vi "TimeLmtDialog.vi"(9 "time(s)":i32=5, 10 "Infoin":string="在这里填写显示的信息内容", 11 "title":string="提示信息") -> ()   [LabVIEW 2011]
panel:
  in  "ok":bool
  out "info":string
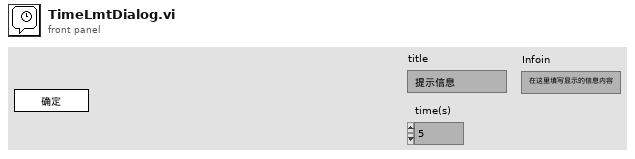
[diagram p1: front panel]
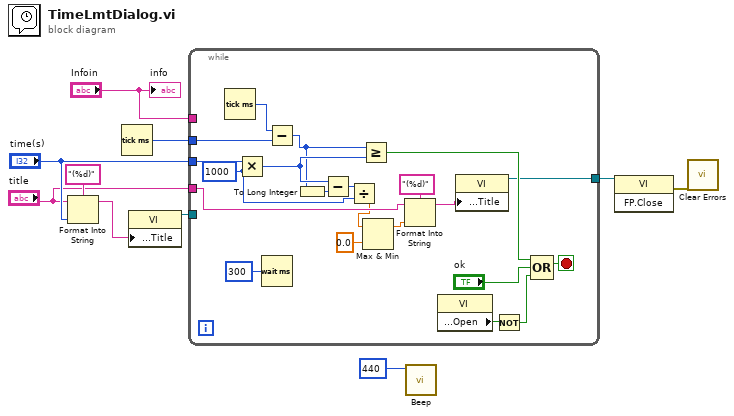
[diagram p0: block diagram]
diagram:
  n1 = Format Into String(format string="(%d)" ("格式字符串"), initial string="title", "time(s)") -> (resulting string=w6:string)  [unwired: 1 in, 1 out]
  n2 = Tick Count (ms)() -> (millisecond timer value=w4:u32)
  n3 = property class="VI"("Front Panel.Title"=w6) -> (reference out=w9:refnum<vi>)  [unwired: 2 in, 1 out]
  n4 = while {
    tunnel: "Infoin" -> [_]
    tunnel: "time(s)" -> [w28]
    tunnel: w9 -> [_]
    tunnel: "title" -> [w20]
    tunnel: w4 -> [w29]
    tunnel: [w13] -> w3
    stop <- w25 stop-if-true
    w21 = 1000 ("y")
    n5 = Tick Count (ms)() -> (millisecond timer value=w30:u32)
    n6 = Multiply(x=w28, y=w21) -> (x*y=w24:i32)
    n7 = Wait (ms)(milliseconds to wait=u32 300 ("等待时间（毫秒）")) -> ()  [unwired: 1 out]
    n8 = Subtract(x=w30, y=w29) -> (x-y=w23:u32)
    n9 = To Long Integer(number=w23) -> (32bit integer=w14:i32)
    n10 = Subtract(x=w24, y=w14) -> (x-y=w22:i32)
    n11 = Divide(x=w22, y=w21) -> (x/y=w17:dbl)
    n12 = Greater Or Equal?(x=w23, y=w24) -> (x >= y?=w26:bool)
    n13 = Max & Min(x=w17, y=0.0) -> (max(x,y)=w15:dbl)  [unwired: 1 out]
    n14 = Format Into String(format string="(%d)" ("格式字符串"), initial string=w20, w15) -> (resulting string=w18:string)  [unwired: 1 in, 1 out]
    n15 = property class="VI"() -> ("Front Panel.Open"=w12:bool)  [unwired: 2 in, 2 out]
    n16 = property class="VI"("Front Panel.Title"=w18) -> (reference out=w13:refnum<vi>)  [unwired: 2 in, 1 out]
    n17 = Not(x=w12) -> (.not. x?=w11:bool)
    n18 = Compound Arithmetic op=OR(w26, "ok", w11) -> (w25:bool)
  }
  n19 = call <vilib>:"Beep.vi"("frequency (Hz)"=u32 440) -> ()  [unwired: 11 in]
  n20 = invoke class="VI" method="FP.Close"(reference=w3) -> (error out=w2:errorcluster)  [unwired: 2 in, 2 out]
  n21 = call <vilib>:"Clear Errors.vi"("error in (no error)"=w2) -> ()  [unwired: 6 in, 1 out]
  "info" <- "Infoin"
